vi "Prompted Inputs Unflatten Test Parameters.vi"(9 "error in (no error)":errorcluster, 10 "Parameter String":string) -> (1 "error out":errorcluster, 2 "Prompted Inputs Test Parameters":T2, 5 "Test Version":string)   [LabVIEW 2011]
uses:
  TypeDefs/PI Test Parameters.ctl
  TypeDefs/PI Measurement Cluster.ctl
  TypeDefs/PI Limit Parameters.ctl
  TypeDefs/PI Limit Definition.ctl
  TypeDefs/PI Limit Comparison.ctl
  Test Return Parameter.ctl
  TypeDefs/PI Test Parameters v1.0-1.2.ctl
  TypeDefs/PI Test Parameters v1.3.ctl
  TypeDefs/PI Test Parameters v1.4.ctl
  TypeDefs/PI Test Parameters v1.5.ctl
  TypeDefs/PI Test Parameters v1.6.ctl
  TypeDefs/PI Test Parameters v1.7.ctl
panel:
  in  "Return Parameter":T1
  out "Parameter Variant":variant
  in  "Required Instruments":string[](array[string])
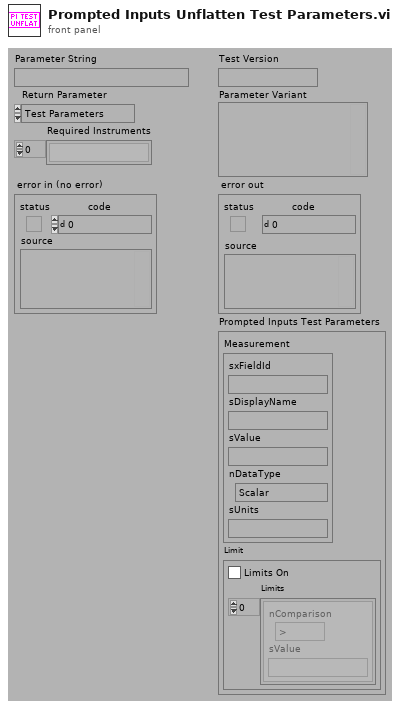
[diagram p1: front panel]
types:
  T1 = typedef "Test Return Parameter.ctl" = enum16{"Test Parameters", "Required Instruments", "Datasheets", "QuickMode"}
  T2 = typedef "PI Test Parameters.ctl" = cluster{"Measurement":T3, "Limit":T4}
  T3 = typedef "PI Measurement Cluster.ctl" = cluster{"sxFieldId":string, "sValue":string, "nDataType":enum16{"Scalar", "Enumeration"}, "sUnits":string, "sDisplayName":string}
  T4 = typedef "PI Limit Parameters.ctl" = cluster{"Limits On":bool, "Limits":T5[]}
  T5 = typedef "PI Limit Definition.ctl" = cluster{"nComparison":T6, "sValue":string}
  T6 = typedef "PI Limit Comparison.ctl" = enum16{">", ">=", "<", "<=", "<>", "="}
  T7 = typedef "PI Test Parameters v1.0-1.2.ctl" = cluster{"Tag":string, "Use Instrument":bool, "Quick Mode":bool, "Blank Screen":bool, "Limits":cluster{"Item":string, "Comparison":enum16{">", ">=", "<", "<="}, "Value":string}[], "Reports":cluster{"Reports to Generate":i32[], "Print Reports":bool}, "Prompted Items":cluster{"Name":string, "Type Value":string, "Key":i32}[]}
  T8 = typedef "PI Test Parameters v1.3.ctl" = cluster{"Tag":string, "Use Instrument":bool, "Quick Mode":bool, "Blank Screen":bool, "Limits":cluster{"Item":string, "Comparison":enum16{">", ">=", "<", "<=", "<>", "="}, "Value":string}[], "Datasheets":cluster{"Datasheets to Generate":i32[], "Print Datasheets":bool}, "Prompted Items":cluster{"Name":string, "Type Value":string, "Key":i32}[]}
  T9 = typedef "PI Test Parameters v1.4.ctl" = cluster{"Limits":cluster{"Item":string, "Comparison":enum16{">", ">=", "<", "<=", "<>", "="}, "Value":string}[], "Datasheets":cluster{"Datasheet to Generate":i32, "Print Datasheets":bool}[], "Prompted Items":cluster{"Name":string, "Type Value":string, "Key":i32}[]}
  T10 = typedef "PI Test Parameters v1.5.ctl" = cluster{"Limits":cluster{"Item":string, "Comparison":enum16{">", ">=", "<", "<=", "<>", "="}, "Value":string}[], "Prompted Inputs":cluster{"Name":string, "Type Value":string, "Key":i32}[]}
  T11 = typedef "PI Test Parameters v1.6.ctl" = cluster{"Measurement":cluster{"Field":string, "Value":string, "Type":enum16{"Scalar", "Enumeration"}}, "Limits":cluster{"Comparison":enum16{">", ">=", "<", "<=", "<>", "="}, "Value":string}[]}
  T12 = typedef "PI Test Parameters v1.7.ctl" = cluster{"Measurement":cluster{"Field":string, "Value":string, "Type":enum16{"Scalar", "Enumeration"}, "Units":string}, "Limit":cluster{"Limits On":bool, "Limits":cluster{"Comparison":enum16{">", ">=", "<", "<=", "<>", "="}, "Value":string}[]}}
  T13 = typedef "Test Datasheets v1.0-4.0.ctl" = cluster{"Datasheet to Generate":i32, "Print Datasheets":bool}[]
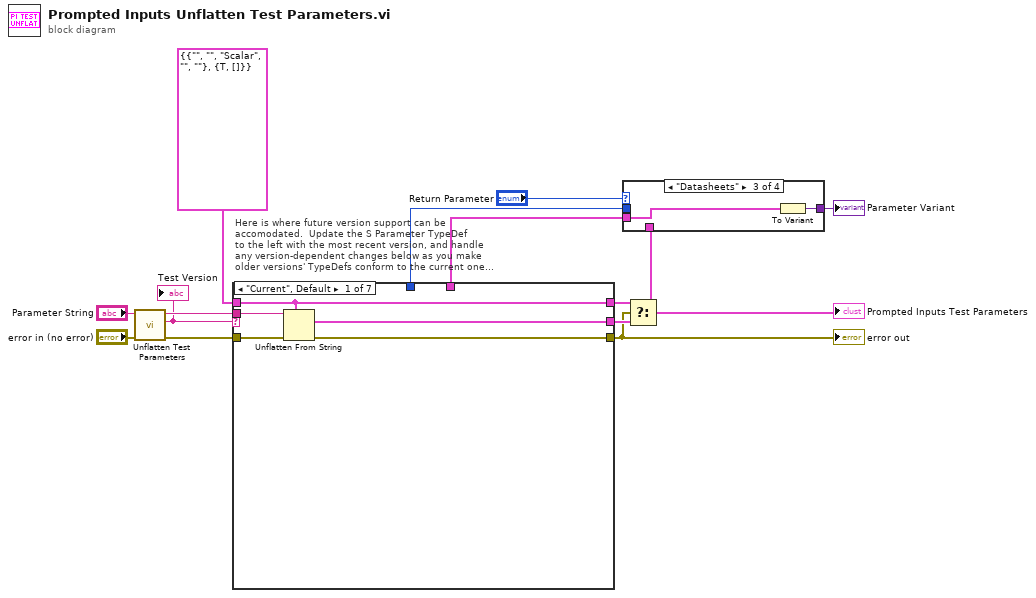
[diagram p0: block diagram]
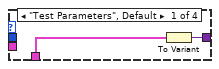
[diagram p2: hidden frame]
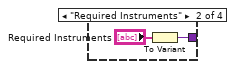
[diagram p3: hidden frame]
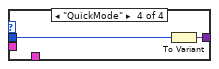
[diagram p4: hidden frame]
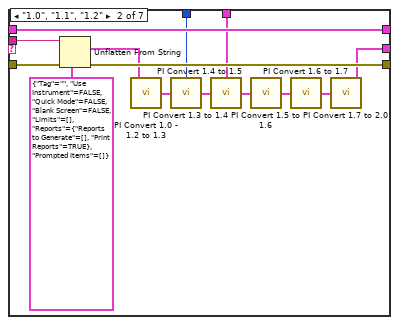
[diagram p5: hidden frame]
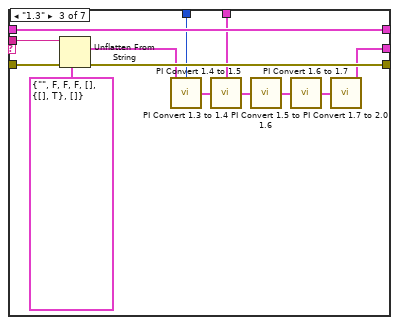
[diagram p6: hidden frame]
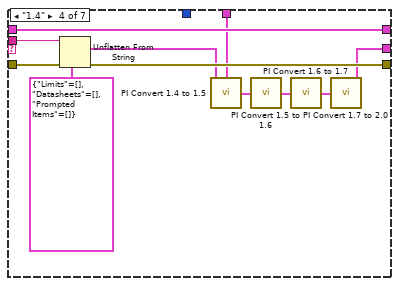
[diagram p7: hidden frame]
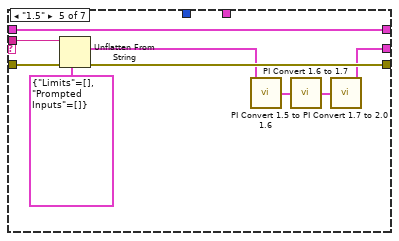
[diagram p8: hidden frame]
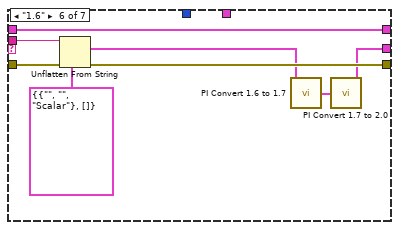
[diagram p9: hidden frame]
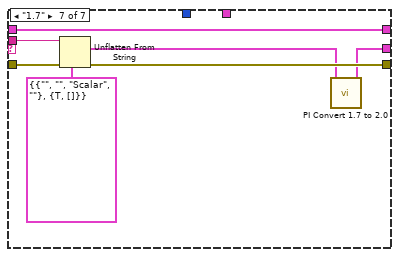
[diagram p10: hidden frame]
diagram:
  # "Here is where future version support can be\naccomodated.  Update the S Parameter TypeDef\nto the left with the most recent version, and handle\nany version-dependent changes below as you make\nolder versions' TypeDefs conform to the current one..."
  n1 = call "Unflatten Test Parameters.vi"("error in (no error)"="error in (no error)", "Flattened Test Parameters with Version (\"\")"="Parameter String") -> ("error out"=w6:errorcluster, "Test Version"=w11:string, "Flat Test Parameters"=w13:string)  [unwired: 3 out]
  "Test Version" <- w11
  n2 = case shown="\"Current\", Default" w11 {
    tunnel: [w18 w20 w34 w47 w58 w67 w76] -> w12
    tunnel: T2 {"Measurement"={"sxFieldId"="", "sValue"="", "nDataType"=enum."Scalar", "sUnits"="", "sDisplayName"=""}, "Limit"={"Limits On"=TRUE, "Limits"=[]}} ("Default Prompt Measurement Configuration\nMost Current Version") -> [w15 w29 w42 w53 w62 w70 w77]
    tunnel: w13 -> [w19 w33 w46 w57 w66 w74 w81]
    tunnel: w6 -> [w17 w32 w45 w56 w65 w73 w80]
    tunnel: [w16 w31 w44 w55 w64 w72 w79] -> w5
    tunnel: [w15 w29 w42 w53 w62 w70 w77] -> w3
    tunnel: [_ w25 w39 w52 _ _ _] -> w1
    tunnel: [_ w24 w38 _ _ _ _] -> w2
    frame "Current", Default {
      n3 = Unflatten From String(type=w15, binary string=w19, error in (no error)=w17) -> (value=w18:T2, error out=w16:errorcluster)  [unwired: 3 out]
    }
    frame "1.0", "1.1", "1.2" {
      n4 = Unflatten From String(type=T7 {"Tag"="", "Use Instrument"=FALSE, "Quick Mode"=FALSE, "Blank Screen"=FALSE, "Limits"=[], "Reports"={"Reports to Generate"=[], "Print Reports"=TRUE}, "Prompted Items"=[]} ("Prompted Inputs Test Parameters"), binary string=w33, error in (no error)=w32) -> (value=w27:T7, error out=w31:errorcluster)  [unwired: 3 out]
      n5 = call "PI Convert 1.0 - 1.2 to 1.3.vi"("Prompted Inputs 1.0 - 1.2 Test Parameters"=w27) -> ("Prompted Inputs 1.3 Test Parameters"=w28:T8)
      n6 = call "PI Convert 1.3 to 1.4.vi"("Prompted Inputs 1.3 Test Parameters"=w28) -> ("QuickMode"=w24:i8, "Prompted Inputs 1.4 Test Parameters"=w26:T9)
      n7 = call "PI Convert 1.4 to 1.5.vi"("Prompted Inputs 1.4 Test Parameters"=w26) -> ("Datasheets"=w25:T13, "Prompted Inputs 1.5 Test Parameters"=w23:T10)
      n8 = call "PI Convert 1.5 to 1.6.vi"("Prompted Inputs 1.5 Test Parameters"=w23) -> ("Prompted Inputs 1.6 Test Parameters"=w22:T11)  [unwired: 1 out]
      n9 = call "PI Convert 1.6 to 1.7.vi"("Prompted Inputs 1.6 Test Parameters"=w22) -> ("Prompted Inputs 1.7 Test Parameters"=w21:T12)  [unwired: 1 out]
      n10 = call "PI Convert 1.7 to 2.0.vi"("Prompted Inputs 1.7 Test Parameters"=w21) -> ("Prompted Inputs 2.0 Test Parameters"=w20:T2)  [unwired: 1 in]
    }
    frame "1.3" {
      n11 = Unflatten From String(type=T8 {"Tag"="", "Use Instrument"=FALSE, "Quick Mode"=FALSE, "Blank Screen"=FALSE, "Limits"=[], "Datasheets"={"Datasheets to Generate"=[], "Print Datasheets"=TRUE}, "Prompted Items"=[]} ("Prompted Inputs Test Parameters"), binary string=w46, error in (no error)=w45) -> (value=w41:T8, error out=w44:errorcluster)  [unwired: 3 out]
      n12 = call "PI Convert 1.3 to 1.4.vi"("Prompted Inputs 1.3 Test Parameters"=w41) -> ("QuickMode"=w38:i8, "Prompted Inputs 1.4 Test Parameters"=w40:T9)
      n13 = call "PI Convert 1.4 to 1.5.vi"("Prompted Inputs 1.4 Test Parameters"=w40) -> ("Datasheets"=w39:T13, "Prompted Inputs 1.5 Test Parameters"=w37:T10)
      n14 = call "PI Convert 1.5 to 1.6.vi"("Prompted Inputs 1.5 Test Parameters"=w37) -> ("Prompted Inputs 1.6 Test Parameters"=w36:T11)  [unwired: 1 out]
      n15 = call "PI Convert 1.6 to 1.7.vi"("Prompted Inputs 1.6 Test Parameters"=w36) -> ("Prompted Inputs 1.7 Test Parameters"=w35:T12)  [unwired: 1 out]
      n16 = call "PI Convert 1.7 to 2.0.vi"("Prompted Inputs 1.7 Test Parameters"=w35) -> ("Prompted Inputs 2.0 Test Parameters"=w34:T2)  [unwired: 1 in]
    }
    frame "1.4" {
      n17 = Unflatten From String(type=T9 {"Limits"=[], "Datasheets"=[], "Prompted Items"=[]} ("Prompted Inputs Test Parameters"), binary string=w57, error in (no error)=w56) -> (value=w51:T9, error out=w55:errorcluster)  [unwired: 3 out]
      n18 = call "PI Convert 1.4 to 1.5.vi"("Prompted Inputs 1.4 Test Parameters"=w51) -> ("Datasheets"=w52:T13, "Prompted Inputs 1.5 Test Parameters"=w50:T10)
      n19 = call "PI Convert 1.5 to 1.6.vi"("Prompted Inputs 1.5 Test Parameters"=w50) -> ("Prompted Inputs 1.6 Test Parameters"=w49:T11)  [unwired: 1 out]
      n20 = call "PI Convert 1.6 to 1.7.vi"("Prompted Inputs 1.6 Test Parameters"=w49) -> ("Prompted Inputs 1.7 Test Parameters"=w48:T12)  [unwired: 1 out]
      n21 = call "PI Convert 1.7 to 2.0.vi"("Prompted Inputs 1.7 Test Parameters"=w48) -> ("Prompted Inputs 2.0 Test Parameters"=w47:T2)  [unwired: 1 in]
    }
    frame "1.5" {
      n22 = Unflatten From String(type=T10 {"Limits"=[], "Prompted Inputs"=[]} ("Prompted Inputs Test Parameters"), binary string=w66, error in (no error)=w65) -> (value=w61:T10, error out=w64:errorcluster)  [unwired: 3 out]
      n23 = call "PI Convert 1.5 to 1.6.vi"("Prompted Inputs 1.5 Test Parameters"=w61) -> ("Prompted Inputs 1.6 Test Parameters"=w60:T11)  [unwired: 1 out]
      n24 = call "PI Convert 1.6 to 1.7.vi"("Prompted Inputs 1.6 Test Parameters"=w60) -> ("Prompted Inputs 1.7 Test Parameters"=w59:T12)  [unwired: 1 out]
      n25 = call "PI Convert 1.7 to 2.0.vi"("Prompted Inputs 1.7 Test Parameters"=w59) -> ("Prompted Inputs 2.0 Test Parameters"=w58:T2)  [unwired: 1 in]
    }
    frame "1.6" {
      n26 = Unflatten From String(type=T11 {"Measurement"={"Field"="", "Value"="", "Type"=enum."Scalar"}, "Limits"=[]} ("Prompted Inputs Test Parameters"), binary string=w74, error in (no error)=w73) -> (value=w69:T11, error out=w72:errorcluster)  [unwired: 3 out]
      n27 = call "PI Convert 1.6 to 1.7.vi"("Prompted Inputs 1.6 Test Parameters"=w69) -> ("Prompted Inputs 1.7 Test Parameters"=w68:T12)  [unwired: 1 out]
      n28 = call "PI Convert 1.7 to 2.0.vi"("Prompted Inputs 1.7 Test Parameters"=w68) -> ("Prompted Inputs 2.0 Test Parameters"=w67:T2)  [unwired: 1 in]
    }
    frame "1.7" {
      n29 = Unflatten From String(type=T12 {"Measurement"={"Field"="", "Value"="", "Type"=enum."Scalar", "Units"=""}, "Limit"={"Limits On"=TRUE, "Limits"=[]}} ("Prompted Inputs Test Parameters"), binary string=w81, error in (no error)=w80) -> (value=w75:T12, error out=w79:errorcluster)  [unwired: 3 out]
      n30 = call "PI Convert 1.7 to 2.0.vi"("Prompted Inputs 1.7 Test Parameters"=w75) -> ("Prompted Inputs 2.0 Test Parameters"=w76:T2)  [unwired: 1 in]
    }
  }
  "error out" <- w5
  n31 = Select(t=w3, s=w5, f=w12) -> (s? t:f=w8:T2)
  "Prompted Inputs Test Parameters" <- w8
  n32 = case shown="\"Datasheets\"" "Return Parameter" {
    tunnel: [w83 w85 w87 w89] -> w9
    tunnel: w8 -> [w82 _ _ _]
    tunnel: w2 -> [_ _ _ w88]
    tunnel: w1 -> [_ _ w86 _]
    frame "Test Parameters", Default {
      n33 = To Variant(anything=w82) -> (Variant=w83:variant)
    }
    frame "Required Instruments" {
      n34 = To Variant(anything="Required Instruments") -> (Variant=w85:variant)
    }
    frame "Datasheets" {
      n35 = To Variant(anything=w86) -> (Variant=w87:variant)
    }
    frame "QuickMode" {
      n36 = To Variant(anything=w88) -> (Variant=w89:variant)
    }
  }
  "Parameter Variant" <- w9
